vi "Que_ENQUE Cmds.vi"(7 "Add To Begining":bool, 8 "Error":errorcluster, 10 "Array":T1[](array[typedef]), 11 "Queue Ref":refnum<queue>) -> (0 "Error Out":errorcluster)   [LabVIEW 2009]
doc: "Enques Commands for Icon editor program"
uses:
  Controls/Cluster/Cluster_Icon Fixer Command Data Set.ctl
  Controls/Enum/ENUM_Icon Fixer Commands.ctl
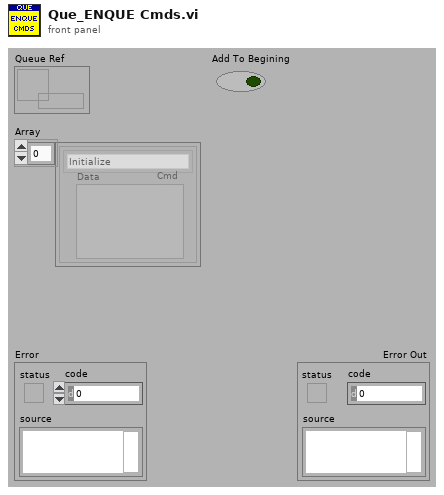
[diagram p1: front panel]
types:
  T1 = typedef "Cluster_Icon Fixer Command Data Set.ctl" = cluster{"Cmd":T2, "Data":variant}
  T2 = typedef "ENUM_Icon Fixer Commands.ctl" = enum16{"NoNe", "Initialize", "Get VI", "Extract Icon", "ReDraw New Icon", "Set Vis Icon", "Save Vi", "Clear String controls", "Set Icon Cluster", "Reset Vis Icon", "Pick Colors", "Upload icon templates", "Download icon templates", "Stop Program", "OCR", "Display Set", "Set Focus", "Set Colors"}
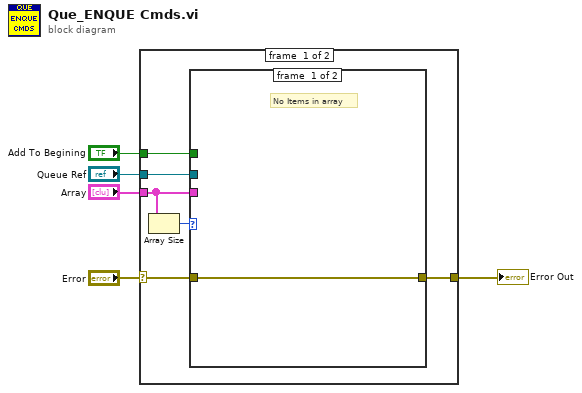
[diagram p0: block diagram]
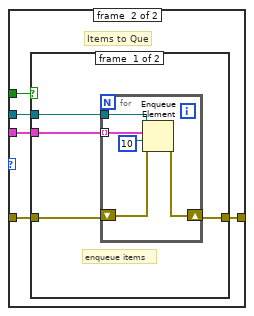
[diagram p2: hidden frame]
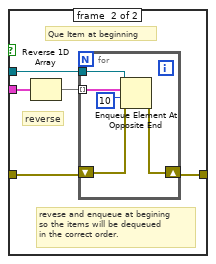
[diagram p3: hidden frame]
diagram:
  n1 = case shown="No Error" "Error" {
    selector: "Error" -> [w6 w37]
    tunnel: "Array" -> [w10 _]
    tunnel: [w9 w37] -> w4
    tunnel: "Queue Ref" -> [w8 _]
    tunnel: "Add To Begining" -> [w7 _]
    frame #0 {
      n2 = Array Size(array=w10) -> (size(s)=w11:i32)
      n3 = case shown="Default" w11 {
        tunnel: w8 -> [_ w17]
        tunnel: [w12 w16] -> w9
        tunnel: w6 -> [w12 w15]
        tunnel: w10 -> [_ w14]
        tunnel: w7 -> [_ w13]
        frame #0 {
          # "No Items in array"
        }
        frame #1 {
          # "Items to Que"
          n4 = case shown="False" w13 {
            tunnel: w17 -> [w21 w31]
            tunnel: [w20 w30] -> w16
            tunnel: w15 -> [w19 w29]
            tunnel: w14 -> [w18 w28]
            frame #0 {
              # "enqueue items"
              n5 = for {
                tunnel: w21 -> [w26]
                shift-right: [w24] -> w20
                shift-left: w19 -> [w25]
                tunnel: w18 -> [w23] mode=indexing
                n6 = Enqueue Element(queue=w26, element=w23, timeout in ms (-1)=10, error in (no error)=w25) -> (error out=w24:errorcluster)  [unwired: 2 out]
              }
            }
            frame #1 {
              # "revese and enqueue at begining\nso the items will be dequeued\nin the correct order."
              # "reverse"
              # "Que Item at beginning"
              n7 = Reverse 1D Array(array=w28) -> (reversed array=w27:T1[])
              n8 = for {
                tunnel: w31 -> [w36]
                shift-right: [w34] -> w30
                shift-left: w29 -> [w35]
                tunnel: w27 -> [w33] mode=indexing
                n9 = Enqueue Element At Opposite End(queue=w36, element=w33, timeout in ms (-1)=10, error in (no error)=w35) -> (error out=w34:errorcluster)  [unwired: 2 out]
              }
            }
          }
        }
      }
    }
    frame #1 {
    }
  }
  "Error Out" <- w4
